vi "parse action report.vi"(8 "error in":errorcluster, 11 "message data":string) -> (0 "error out":errorcluster)   [LabVIEW 2013, in "module execution process.lvlib"]
uses:
  module execution process.lvlib
  command commands to rtexe process.ctl
panel:
  out "command error":errorcluster
  out "commands":T1
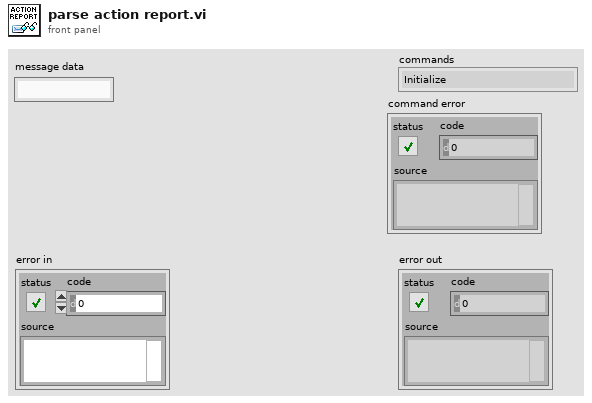
[diagram p1: front panel]
types:
  T1 = typedef "module execution process.lvlib/command commands to rtexe process.ctl" = enum16{"Initialize", "Load from File", "Load from String", "Open All Engines", "Open Single Engine", "Initialize All Engines", "Initialize Single Engine", "Start All", "Start Single", "Pause All", "Pause Single", "Stop All", "Stop Single", "Close All", "Close Single", "Set Safe State All", "Set Safe State Single", "Get Status", "Exit", "Error", "Add Search Paths"}
  T2 = cluster{"command string":string, "command error":errorcluster}
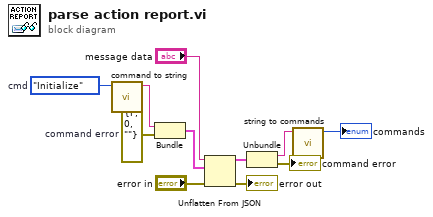
[diagram p0: block diagram]
diagram:
  w4 = errorcluster {"status"=FALSE, "code"=0, "source"=""}  # command error
  w6 = command_commands_to_rtexe_process."Initialize"  # cmd
  n1 = call "command to string.vi"("commands"=w6) -> ("command string"=w5:string)  [unwired: 10 in]
  n2 = Bundle("command string"=w5, "command error"=w4) -> (w3:T2)  [unwired: 1 in]
  n3 = Unflatten From JSON(JSON string="message data", type and defaults=w3, error in (no error)="error in") -> (value=w8:T2, error out=→"error out":errorcluster)  [unwired: 4 in]
  n4 = Unbundle(w8) -> ("command string"=w2:string, "command error"=→"command error":errorcluster)
  n5 = call "string to commands.vi"("command string"=w2) -> ("commands"=→"commands":T1)  [unwired: 9 in, 1 out]
